vi "String_parsing.vi"() -> ()   [LabVIEW 2014]
panel:
  out "V3":i32[](array[numeric])
  out "V2":i32[](array[numeric])
  out "V1":i32[](array[numeric])
  out "unsigned byte array":u8[](array[numeric])
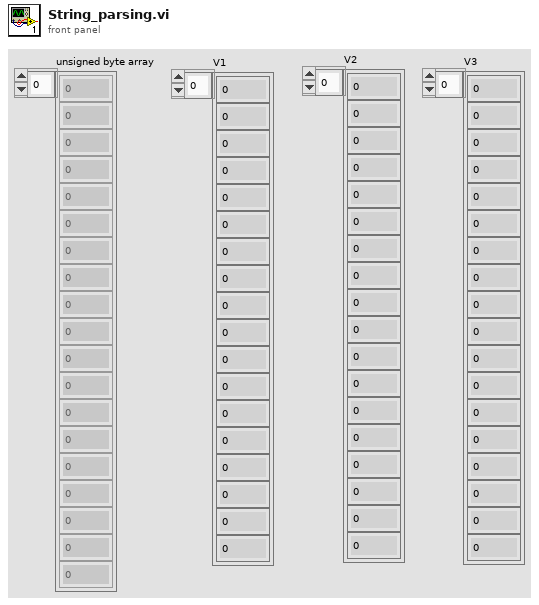
[diagram p1: front panel]
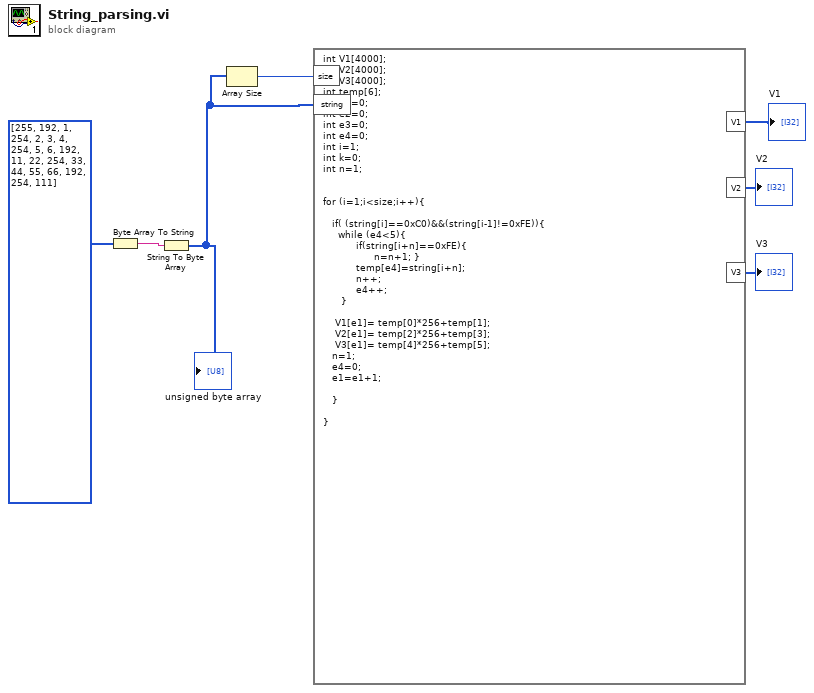
[diagram p0: block diagram]
diagram:
  n1 = Byte Array To String(unsigned byte array=u8[] [255, 192, 1, 254, 2, 3, 4, 254, 5, 6, 192, 11, 22, 254, 33, 44, 55, 66, 192, 254, 111]) -> (string=w6:string)
  n2 = String To Byte Array(string=w6) -> (unsigned byte array=w4:u8[])
  "unsigned byte array" <- w4
  n3 = Array Size(array=w4) -> (size(s)=w3:i32)
  n4 = formula code="int V1[4000];\nint V2[4000];\nint V3[4000];\nint temp[6];\nint e1=0;\nint e2=0;\nint e3=0;\nint e4=0;\nint i=1;\nint k=0;\nint n=1;\n\n\nfor (i=1;i<size;i++){\n\n   if( (string[i]==0xC0)&&(string[i-1]!=0xFE)){ \n     while (e4<5){\n           if(string[i+n]==0xFE){\n                 n=n+1; }\n           temp[e4]=string[i+n];\n           n++; \n           e4++;\n      }\n   \n    V1[e1]= temp[0]*256+temp[1];\n    V2[e1]= temp[2]*256+temp[3];\n    V3[e1]= temp[4]*256+temp[5];\n   n=1;\n   e4=0;\n   e1=e1+1;\n   \n   }\n\n}"("string"=w4, "size"=w3) -> ("V1"=→"V1":i32[], "V2"=→"V2":i32[], "V3"=→"V3":i32[])
